vi "Custom_Create_VI_BlockDiagram_Images.vi"(6 "Printing:Custom Diagram Repeat?":bool, 7 "Printing:Custom Diagram Hidden?":bool, 8 "error in (no error)":errorcluster, 9 "Image Depth":i32=24, 10 "Image Format (jpeg)":enum32{"PNG", "JPEG", "GIF"}(ring)=enum."JPEG", 11 "VI":refnum<vi>) -> (0 "error out":errorcluster, 3 "Paths to images":path[](array[path]))   [LabVIEW 2019]
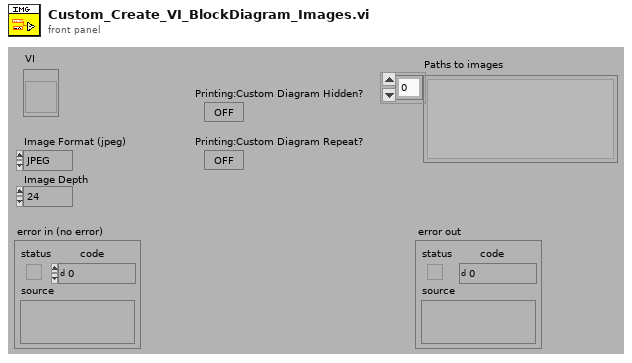
[diagram p1: front panel]
types:
  T1 = cluster{"Printing:Custom All Controls?":bool, "Printing:Custom Connector?":bool, "Printing:Custom Control Descriptions?":bool, "Printing:Custom Control Types?":bool, "Printing:Custom Controls?":bool, "Printing:Custom Description?":bool, "Printing:Custom Diagram Hidden?":bool, "Printing:Custom Diagram Repeat?":bool, "Printing:Custom Diagram?":bool, "Printing:Custom Hierarchy?":bool, "Printing:Custom History?":bool, "Printing:Custom Panel Border?":bool, "Printing:Custom Panel?":bool, "Printing:Custom SubVIs?":bool}
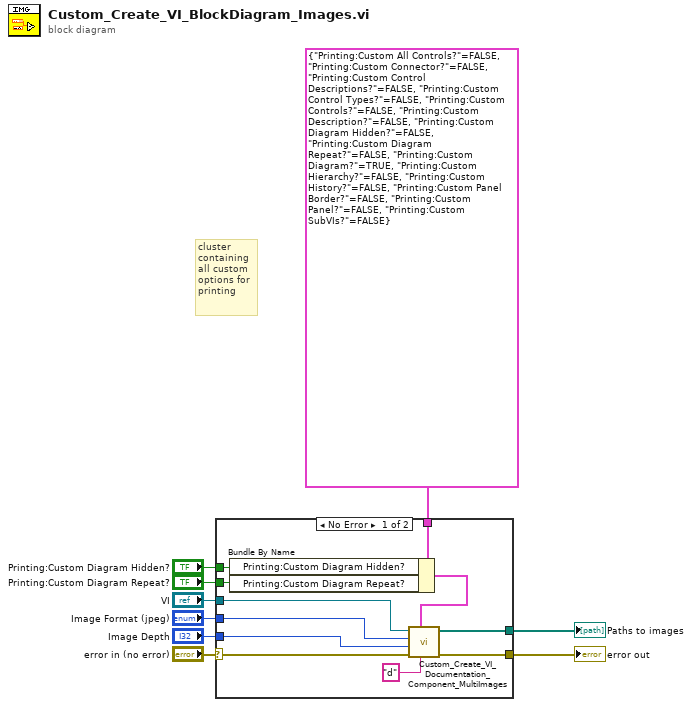
[diagram p0: block diagram]
diagram:
  # "cluster\ncontaining\nall custom\noptions for\nprinting"
  n1 = case shown="No Error" "error in (no error)" {
    selector: "error in (no error)" -> [w11 w21]
    tunnel: "VI" -> [w20 _]
    tunnel: "Image Format (jpeg)" -> [w19 _]
    tunnel: "Image Depth" -> [w18 _]
    tunnel: [w17 w21] -> w6
    tunnel: T1 {"Printing:Custom All Controls?"=FALSE, "Printing:Custom Connector?"=FALSE, "Printing:Custom Control Descriptions?"=FALSE, "Printing:Custom Control Types?"=FALSE, "Printing:Custom Controls?"=FALSE, "Printing:Custom Description?"=FALSE, "Printing:Custom Diagram Hidden?"=FALSE, "Printing:Custom Diagram Repeat?"=FALSE, "Printing:Custom Diagram?"=TRUE, "Printing:Custom Hierarchy?"=FALSE, "Printing:Custom History?"=FALSE, "Printing:Custom Panel Border?"=FALSE, "Printing:Custom Panel?"=FALSE, "Printing:Custom SubVIs?"=FALSE} ("Content Options") -> [w16 _]
    tunnel: "Printing:Custom Diagram Hidden?" -> [w14 _]
    tunnel: "Printing:Custom Diagram Repeat?" -> [w13 _]
    tunnel: [w12 _] -> w2
    frame No Error {
      n2 = Bundle By Name(cluster=w16, "Printing:Custom Diagram Hidden?"=w14, "Printing:Custom Diagram Repeat?"=w13) -> (w15:T1)
      n3 = call "Custom_Create_VI_Documentation_Component_MultiImages.vi"("special chars in file path of image"="d", "Content Options"=w15, "error in (no error)"=w11, "Image Depth"=w18, "Image Format (jpeg)"=w19, "VI"=w20) -> ("error out"=w17:errorcluster, "Paths to images"=w12:path[])  [unwired: 4 in]
    }
    frame Error {
    }
  }
  "error out" <- w6
  "Paths to images" <- w2
